vi "Acquire data continuously.vi"() -> ()   [LabVIEW 2020]
uses:
  <vilib>/DAQmx/read.llb/DAQmx Read (Analog 1D Wfm NChan NSamp).vi
  <vilib>/Analysis/baseanly.llb/Mean (DBL).vi
  <vilib>/DAQmx/create/channels.llb/DAQmx Create Channel (AI-Voltage-Basic).vi
  <vilib>/DAQmx/configure/timing.llb/DAQmx Timing (Sample Clock).vi
  <vilib>/DAQmx/configure/task.llb/DAQmx Configure Logging (TDMS).vi
  <vilib>/DAQmx/miscellaneous.llb/DAQmx Fill In Error Info.vi
  <resource>/objmgr/daqmx.rc
  <vilib>/Analysis/NI_AALBase.lvlib
panel:
  out "mean":dbl format="%0.4f"
  out "error out":errorcluster
  out "Waveform Graph":waveform(dbl)[](graph)
  in  "Stop":bool
  in  "Number of Samples":i32=100
  in  "TDMS File Path":path
  in  "Sample Rate":dbl=1000.0
  in  "Sample Clock Source":tag="OnboardClock"
  in  "Terminal Configuration":i32(ring)=-1 items=["default"=-1, "RSE"=10083, "NRSE"=10078, "Differential"=10106, "Pseudodifferential"=12529]
  in  "Max Voltage":dbl=5.0
  in  "Min Voltage":dbl=-5.0
  in  "Physical Channel":tag="Dev1/ai0"
  out "Actual Sample Rate":dbl=1000.0 format="%0.2f"
  in  "Logging Mode":i32(ring)=10231 items=["Off"=10231, "Log and Read"=15842]
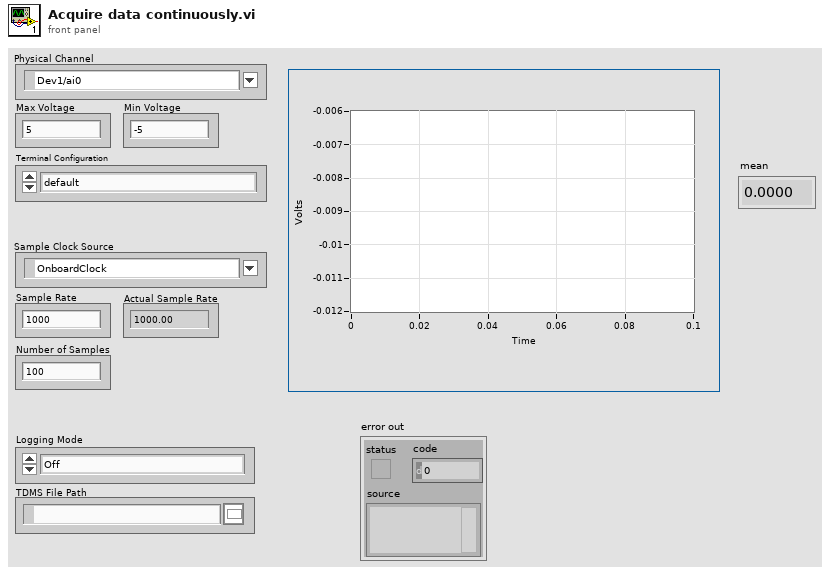
[diagram p1: front panel]
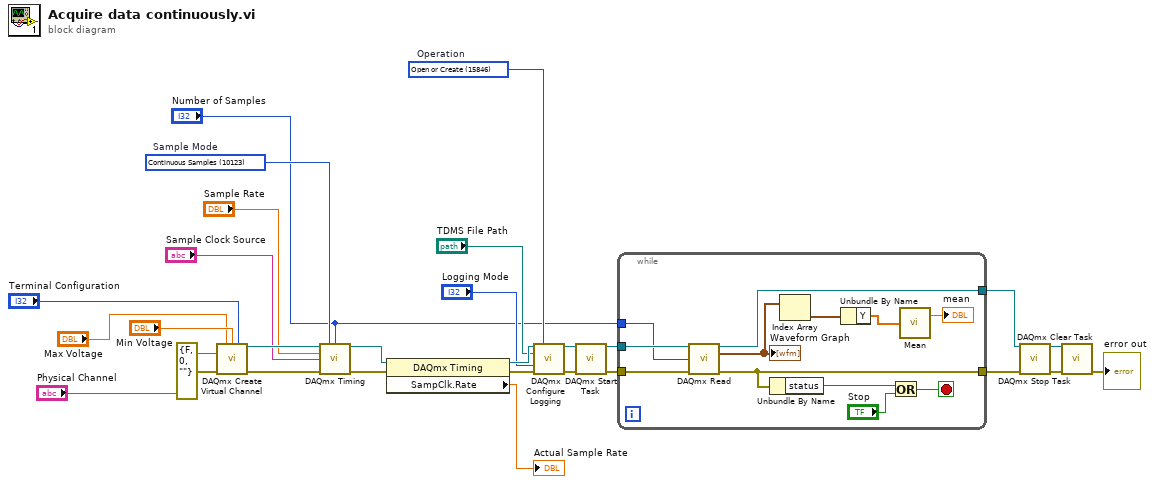
[diagram p0: block diagram]
diagram:
  w21 = 15846 items=["Open"=10437, "Open or Create"=15846, "Create or Replace"=15847, "Create"=15848]  # Operation
  w26 = 10123 items=["Finite Samples"=10178, "Continuous Samples"=10123, "Hardware Timed Single Point"=12522]  # Sample Mode
  n1 = call-poly <vilib>:"DAQmx Create Virtual Channel.vi"("maximum value"="Max Voltage", "minimum value"="Min Voltage", "input terminal configuration"="Terminal Configuration", "physical channels"="Physical Channel", "error in"=errorcluster {"status"=FALSE, "code"=0, "source"=""}) -> ("task out"=w24:refnum<k21>, "error out"=w25:errorcluster)  [unwired: 9 in]
  n2 = call-poly <vilib>:"DAQmx Timing.vi"("task/channels in"=w24, "sample mode"=w26, "samples per channel"="Number of Samples", "rate"="Sample Rate", "source"="Sample Clock Source", "error in"=w25) -> ("task out"=w28:refnum<k21>, "error out"=w27:errorcluster)  [unwired: 8 in]
  n3 = property class="DAQmx Timing"(reference=w28, error in=w27) -> (reference out=w23:refnum<k21>, error out=w22:errorcluster, "SampClk.Rate"=→"Actual Sample Rate":dbl)
  n4 = call-poly <vilib>:"DAQmx Configure Logging.vi"("task/channels in"=w23, "operation"=w21, "file path"="TDMS File Path", "logging mode"="Logging Mode", "error in"=w22) -> ("task out"=w3:refnum<k21>, "error out"=w4:errorcluster)  [unwired: 9 in]
  n5 = call <vilib>:"DAQmx Start Task.vi"("task/channels in"=w3, "error in"=w4) -> ("task out"=w20:refnum<k21>, "error out"=w19:errorcluster)  [unwired: 12 in]
  n6 = while {
    tunnel: w20 -> [w40]
    tunnel: w19 -> [w39]
    tunnel: [w38] -> w8
    tunnel: [w36] -> w7
    tunnel: "Number of Samples" -> [w33]
    stop <- w34 stop-if-true
    n7 = call-poly <vilib>:"DAQmx Read.vi"("task/channels in"=w40, "number of samples per channel"=w33, "error in"=w39) -> ("task out"=w38:refnum<k21>, "data"=w32:waveform(dbl)[], "error out"=w36:errorcluster)  [unwired: 10 in]
    "Waveform Graph" <- w32
    n8 = Unbundle By Name(w36) -> ("status"=w35:bool)
    n9 = Index Array(array=w32) -> (element=w31:waveform(dbl))  [unwired: 1 in]
    n10 = Unbundle By Name(w31) -> ("Y"=w30:dbl[])
    n11 = Or(x=w35, y="Stop") -> (x .or. y?=w34:bool)
    n12 = call-poly <vilib>:"Mean.vi"("X"=w30) -> ("mean"=→"mean":dbl)  [unwired: 1 out]
  }
  n13 = call <vilib>:"DAQmx Stop Task.vi"("task/channels in"=w8, "error in"=w7) -> ("task out"=w5:refnum<k21>, "error out"=w6:errorcluster)  [unwired: 12 in]
  n14 = call <vilib>:"DAQmx Clear Task.vi"("task in"=w5, "error in"=w6) -> ("error out"=→"error out":errorcluster)  [unwired: 13 in]
